vi "SourceInfo.vi"(6 "error in (no error)":errorcluster, 9 "Source":string) -> (0 "error out":errorcluster, 3 "Source out":string, 4 "SourceStatus":T1)   [LabVIEW 2009]
uses:
  Controls/SourceStatus.ctl
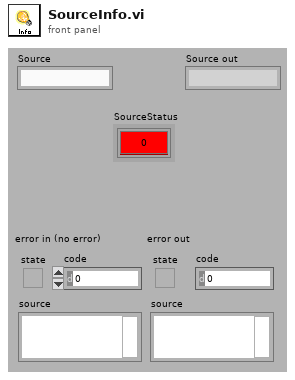
[diagram p1: front panel]
types:
  T1 = typedef "SourceStatus.ctl" = cluster{"Managed?":bool, "Intensity":i32}
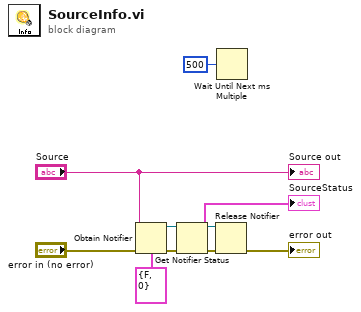
[diagram p0: block diagram]
diagram:
  n1 = Obtain Notifier(name (unnamed)="Source", notification data type=T1 {"Managed?"=FALSE, "Intensity"=0} ("Source Status"), error in (no error)="error in (no error)") -> (notifier out=w7:refnum<notifier>, error out=w2:errorcluster)  [unwired: 1 in, 1 out]
  n2 = Get Notifier Status(notifier=w7, error in (no error)=w2) -> (notifier out=w9:refnum<notifier>, current notification=→"SourceStatus":T1, error out=w8:errorcluster)  [unwired: 2 out]
  n3 = Release Notifier(notifier=w9, error in (no error)=w8) -> (error out=→"error out":errorcluster)  [unwired: 3 out]
  n4 = Wait Until Next ms Multiple(millisecond multiple=u32 500 ("n millisecondes")) -> ()  [unwired: 1 out]
  "Source out" <- "Source"
